vi "iradon_only.vi"() -> ()   [LabVIEW 2018]
panel:
  out "x/y":dbl[][](array[numeric])
  in  "2-D Array of Real":dbl[][](array[numeric])
  in  "N_det":dbl=40.0
  in  "N_rot":dbl=40.0
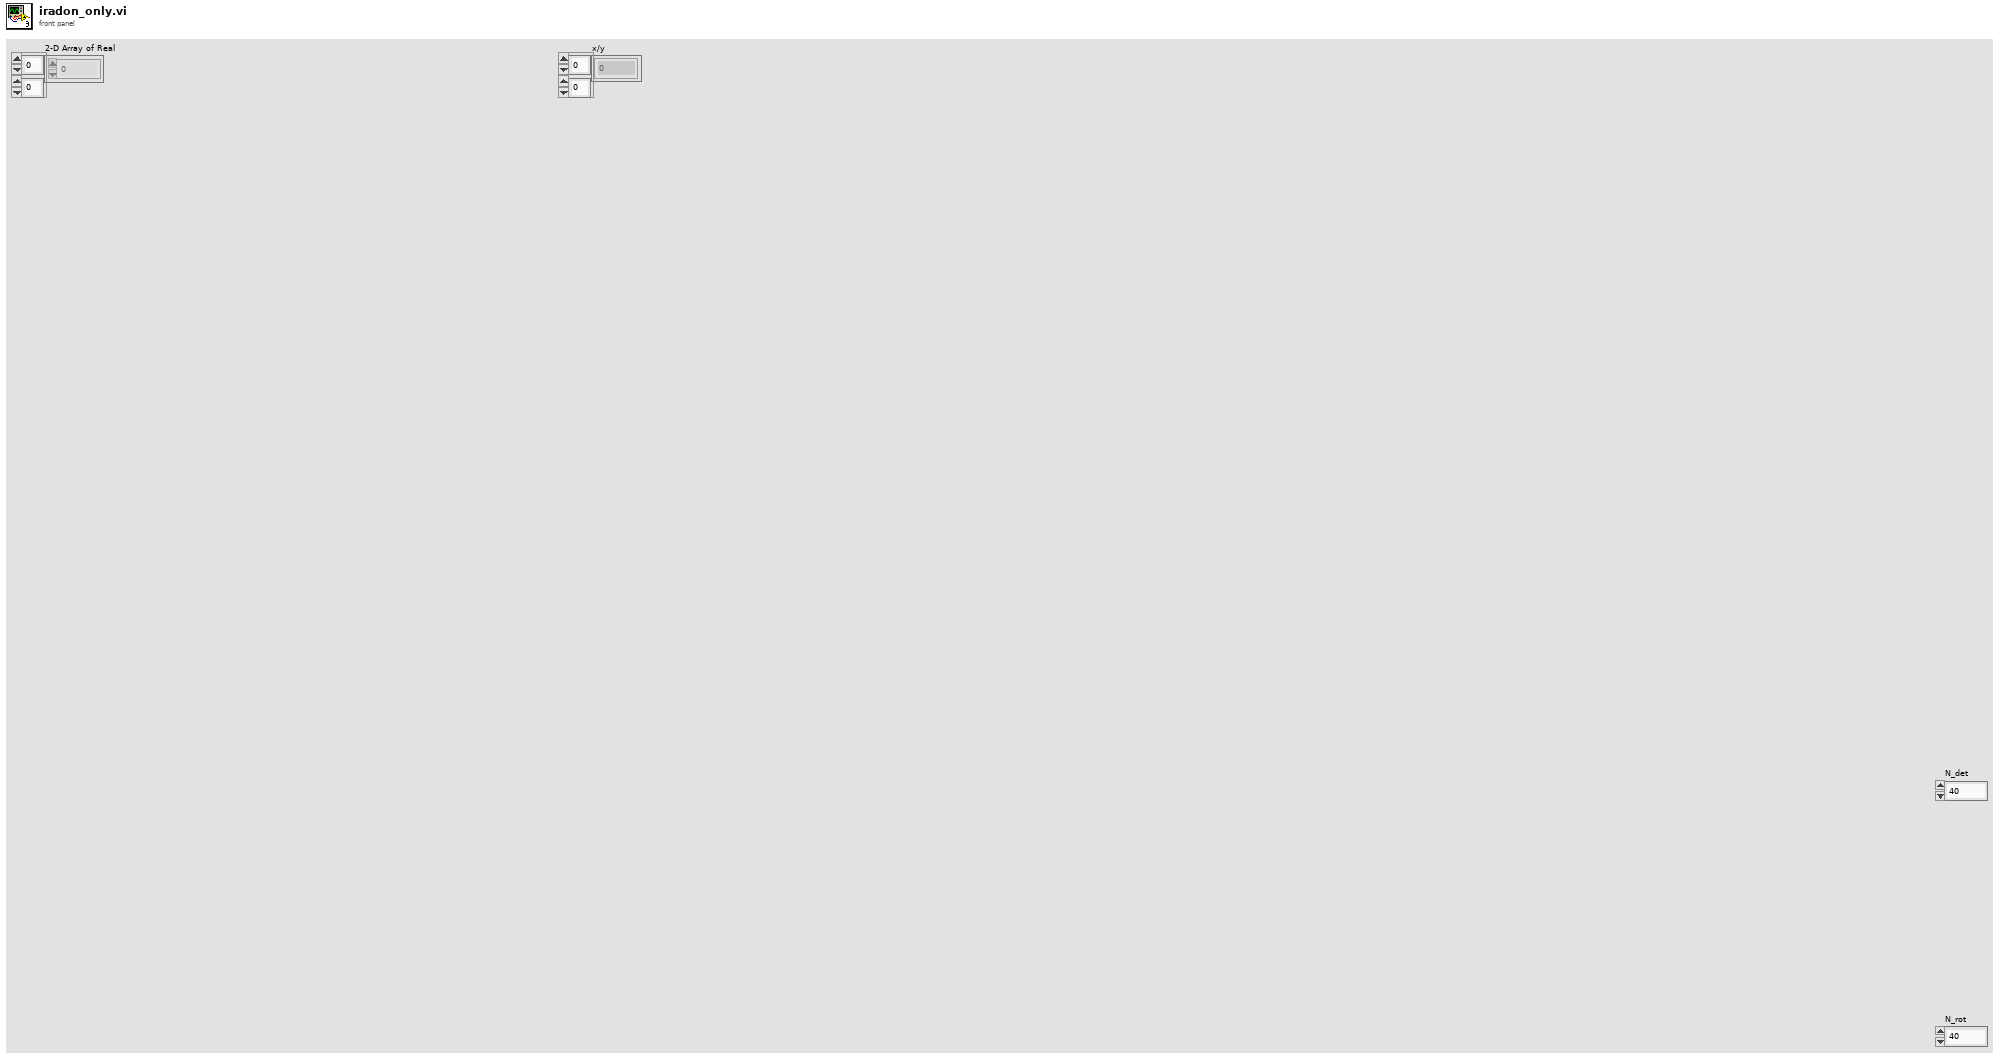
[diagram p1: front panel]
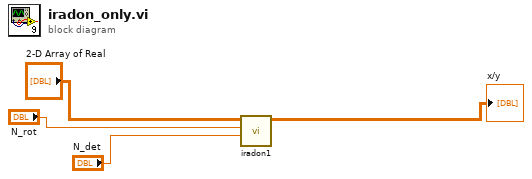
[diagram p0: block diagram]
diagram:
  n1 = call "iradon1.vi"("N_det"="N_det", "N_rot"="N_rot", "2-D Array of Real"="2-D Array of Real") -> ("x/y"=→"x/y":dbl[][])  [unwired: 8 in]
